vi "CaseTimer.vi"(8 "CaseTime":u32[](array[numeric])=[1000, 1000, 1000, 1000, 1000, 1000, 1000], 11 "ElapsedTime":i32=6000) -> (3 "CaseNumber":i32)   [LabVIEW 2017]
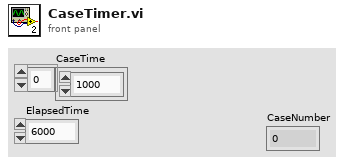
[diagram p1: front panel]
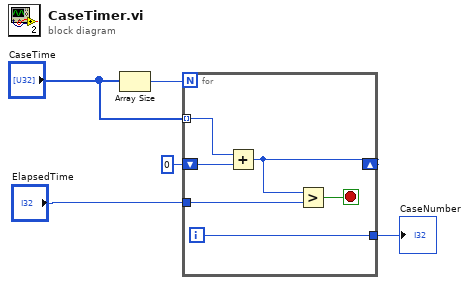
[diagram p0: block diagram]
diagram:
  n1 = Array Size(array="CaseTime") -> (size(s)=w5:i32)
  n2 = for {
    N: w5 -> [_]
    shift-right: [w7] -> _
    shift-left: u32 0 -> [w10]
    tunnel: "ElapsedTime" -> [w6]
    tunnel: "CaseTime" -> [w11] mode=indexing
    tunnel: [w9] -> w4
    i -> [w9]
    stop <- w8 stop-if-true
    n3 = Add(x=w11, y=w10) -> (x+y=w7:u32)
    n4 = Greater?(x=w7, y=w6) -> (0:w8:bool)
  }
  "CaseNumber" <- w4
